vi "MGI Get Custom Error Codes.vi"(11 "MGI Error Reporter Base In":refnum<class "MGI Error Reporter Base.lvclass">) -> (1 "Custom Name[]":string[](array[string]), 2 "Custom Code[]":i32[](array[numeric]))   [LabVIEW 2016, in "MGI Error Reporter Base.lvclass"]
doc: "Output the custom error codes defined for the Error Reporter.\n\nAuthored by Shawn Walpole\nsupport@mooregoodideas.com\nwww.mooregoodideas.com\n\nCopyright (c) 2013, Moore Good Ideas, Inc.\n\nAll rights reserved.\n\nRedistribution and use in source and binary forms, with or without modification, are permitted provided that the following conditions are met:\n\n * Redistributions of source code must retain the above copyright notice, this list of conditions and the following disclaimer.\n * Redistributions in binary form must reproduce the above copyright notice, this list of conditions and the following disclaimer in the documentation and/or other materials provided with the distribution.\n * Neither the name of Moore Good Ideas, Inc. nor the names of its contributors may be used to endorse or promote products derived from this software without specific prior written permission.\n\nTHIS SOFTWARE IS PROVIDED BY THE COPYRIGHT HOLDERS AND CONTRIBUTORS \"AS IS\" AND ANY EXPRESS OR IMPLIED WARRANTIES, INCLUDING, BUT NOT LIMITED TO, THE IMPLIED WARRANTIES OF MERCHANTABILITY AND FITNESS FOR A PARTICULAR PURPOSE ARE DISCLAIMED. IN NO EVENT SHALL THE COPYRIGHT OWNER OR CONTRIBUTORS BE LIABLE FOR ANY DIRECT, INDIRECT, INCIDENTAL, SPECIAL, EXEMPLARY, OR CONSEQUENTIAL DAMAGES (INCLUDING, BUT NOT LIMITED TO, PROCUREMENT OF SUBSTITUTE GOODS OR SERVICES; LOSS OF USE, DATA, OR PROFITS; OR BUSINESS INTERRUPTION) HOWEVER CAUSED AND ON ANY THEORY OF LIABILITY, WHETHER IN CONTRACT, STRICT LIABILITY, OR TORT (INCLUDING NEGLIGENCE OR OTHERWISE) ARISING IN ANY WAY OUT OF THE USE OF THIS SOFTWARE, EVEN IF ADVISED OF THE POSSIBILITY OF SUCH DAMAGE."
uses:
  <userlib>/_MGI/Error Reporter/MGI Error Reporter Base/MGI Error Reporter Base.lvclass
  <userlib>/_MGI/Error Reporter/MGI Error Reporter Base/MGI Error Reporter Base.lvclass/MGI Error Reporter Base.ctl
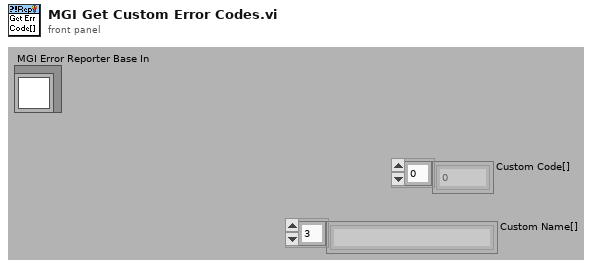
[diagram p1: front panel]
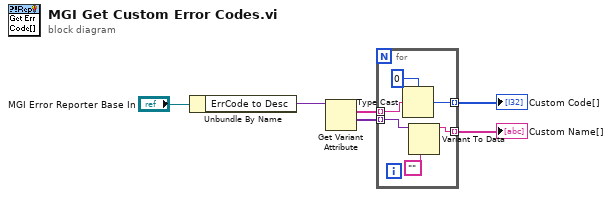
[diagram p0: block diagram]
diagram:
  n1 = Unbundle By Name("MGI Error Reporter Base In") -> ("ErrCode to Desc"=w2:variant)
  n2 = Get Variant Attribute(Variant=w2) -> (names=w6:string[], values=w5:variant[])  [unwired: 1 in, 4 out]
  n3 = for {
    tunnel: [w12] -> w3 mode=indexing
    tunnel: w6 -> [w10] mode=indexing
    tunnel: w5 -> [w11] mode=indexing
    tunnel: [w8] -> w4 mode=indexing
    n4 = Type Cast(type=0, x=w10) -> (*(type *) &x=w8:i32)
    n5 = Variant To Data(type="", Variant=w11) -> (data=w12:string)  [unwired: 1 in, 1 out]
  }
  "Custom Name[]" <- w3
  "Custom Code[]" <- w4
